vi "liblinear_cross_validation.vi"(8 "error in (no error)":errorcluster, 9 "nr_fold":i32, 10 "parameters":T3={"solver_type"=0, "eps"=0.01, "C"=1.0, "weight_label"=[], "weight"=[], "p"=0.1} {"solver_type" items=["L2R_LR"=0, "L2R_L2LOSS_SVC_DUAL"=1, "L2R_L2LOSS_SVC"=2, "L2R_L1LOSS_SVC_DUAL"=3, "MCSVM_CS"=4, "L1R_L2LOSS_SVC"=5, "L1R_LR"=6, "L2R_LR_DUAL"=7, "L2R_L2LOSS_SVR"=11, "L2R_L2LOSS_SVR_DUAL"=12, "L2R_L1LOSS_SVR_DUAL"=13]}, 11 "problem":T1={"y"=[], "x"=[], "bias"=-1.0}) -> (0 "error out":errorcluster, 3 "target":dbl[](array[numeric]))   [LabVIEW 2014]
uses:
  Controls/liblinear_parameter.ctl
  Controls/liblinear_solver.ctl
  Controls/liblinear_problem.ctl
  Libsvm Wrapper/Controls/svm_node.ctl
  <vilib>/oysstu/LVLibSVM/bin/x64/LVLibSVM.dll
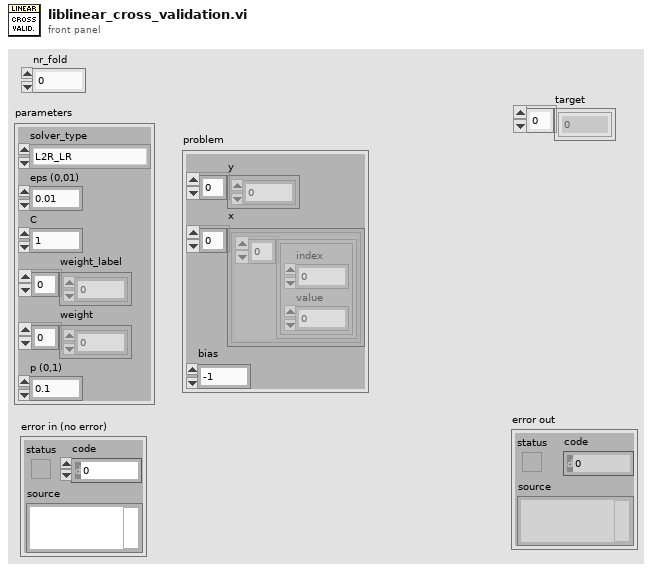
[diagram p1: front panel]
types:
  T1 = typedef "liblinear_problem.ctl" = cluster{"y":dbl[], "x":cluster{T2[]}[], "bias":dbl}
  T2 = typedef "svm_node.ctl" = cluster{"index":i32, "value":dbl}
  T3 = typedef "liblinear_parameter.ctl" = cluster{"solver_type":T4, "eps":dbl, "C":dbl, "weight_label":i32[], "weight":dbl[], "p":dbl}
  T4 = typedef "liblinear_solver.ctl" = u32
  T5 = typedef "liblinear_problem_padded.ctl" = cluster{"y":dbl[], "x":cluster{T6[]}[], "bias":dbl}
  T6 = typedef "liblinear_node_padded.ctl" = cluster{"index":i32, "padding":i32, "value":dbl}
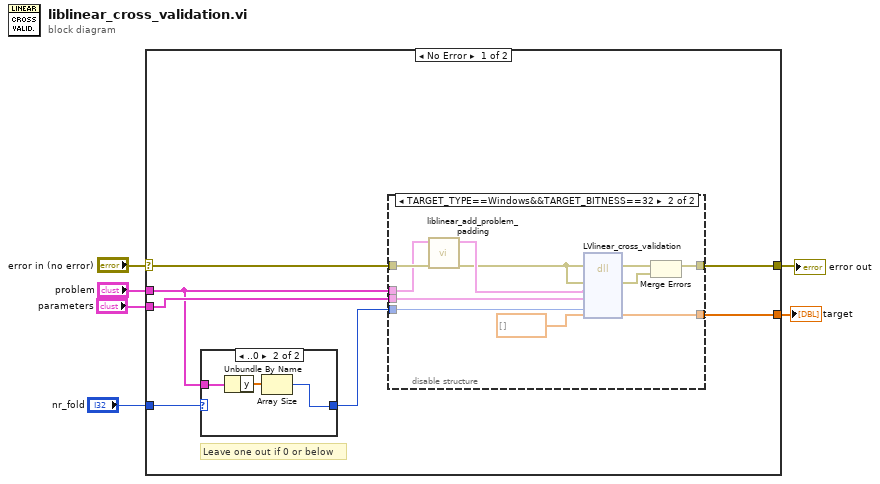
[diagram p0: block diagram]
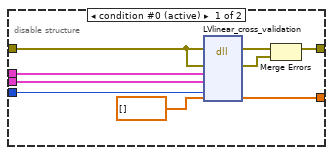
[diagram p2: hidden frame]
diagram:
  n1 = case shown="No Error" "error in (no error)" {
    selector: "error in (no error)" -> [w12 w38]
    tunnel: [w13 w38] -> w6
    tunnel: "nr_fold" -> [w8 _]
    tunnel: "problem" -> [w9 _]
    tunnel: "parameters" -> [w11 _]
    tunnel: [w10 _] -> w1
    frame No Error {
      # "Leave one out if 0 or below"
      n2 = case shown="..0" w8 {
        selector: w8 -> [w34 _]
        tunnel: w9 -> [_ w37]
        tunnel: [w34 w35] -> w7
        frame Default {
        }
        frame ..0 {
          n3 = Unbundle By Name(w37) -> ("y"=w36:dbl[])
          n4 = Array Size(array=w36) -> (size(s)=w35:i32)
        }
      }
      n5 = disable-structure shown="TARGET_TYPE==Windows&&TARGET_BITNESS==32" {
        disable-tunnel: [w21 w32] -> w13
        disable-tunnel: w12 -> [w20 w26]
        disable-tunnel: w11 -> [w18 w30]
        disable-tunnel: [w16 w28] -> w10
        disable-tunnel: w9 -> [w15 w25]
        disable-tunnel: w7 -> [w14 w27]
        frame condition #0 (active) {
          n6 = dll-call lib="C:/Program Files/National Instruments/LabVIEW 2014/vi.lib/oysstu/LVLibSVM/bin/x64/LVLibSVM.dll" fn="LVlinear_cross_validation"(error in=w20, "lvErr"=w20, "prob_in"=w15, "param_in"=w18, "nr_fold"=w14, "target_out"=dbl[] []) -> (error out=w22:errorcluster, "lvErr"=w19:errorcluster, "target_out"=w16:dbl[])  [unwired: 6 in, 1 out]
          n7 = Merge Errors(w22, w19) -> (w21:errorcluster)
        }
        frame condition #1 {
          n8 = call "liblinear_add_problem_padding.vi"("error in (no error)"=w26, "problem"=w25) -> ("error out"=w23:errorcluster, "problem padded"=w24:T5)  [unwired: 8 in]
          n9 = dll-call lib="C:/Program Files/National Instruments/LabVIEW 2014/vi.lib/oysstu/LVLibSVM/bin/x64/LVLibSVM.dll" fn="LVlinear_cross_validation"(error in=w23, "lvErr"=w23, "prob_in"=w24, "param_in"=w30, "nr_fold"=w27, "target_out"=dbl[] []) -> (error out=w33:errorcluster, "lvErr"=w31:errorcluster, "target_out"=w28:dbl[])  [unwired: 6 in, 1 out]
          n10 = Merge Errors(w33, w31) -> (w32:errorcluster)
        }
      }
    }
    frame Error {
    }
  }
  "error out" <- w6
  "target" <- w1
